vi "MakeTopFolder.vi"(8 "error in (no error)":errorcluster, 10 "Comment":string, 11 "Loggers":path=path "C:/Users/dpl/OneDrive - Aberystwyth University/Documents/LabVIEW Data/TestExecutive/TestData") -> (0 "error out":errorcluster, 2 "TopFolderPrefix":string, 3 "TestFolderPath":path)   [LabVIEW 2024]
uses:
  <userlib>/_OpenG.lib/file/file.llb/openg_file.lvlib
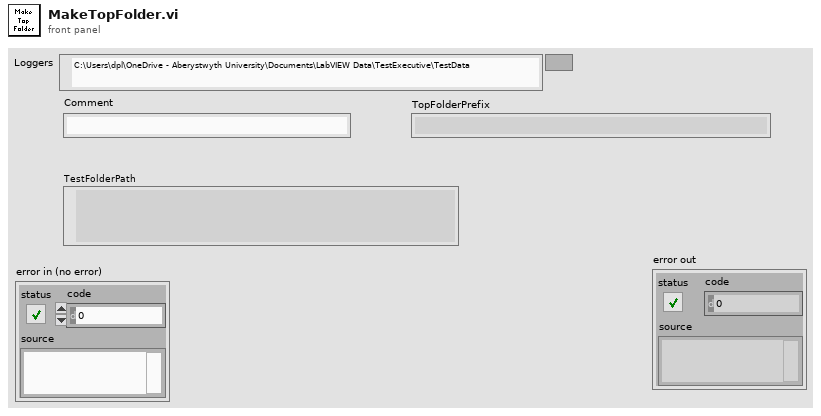
[diagram p1: front panel]
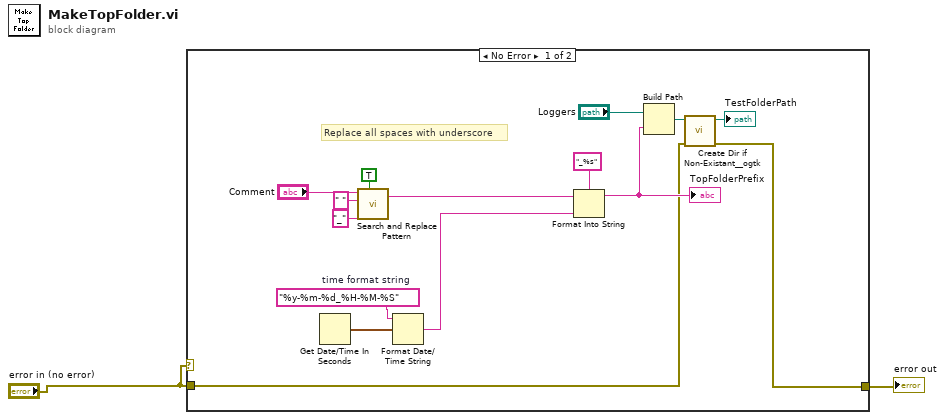
[diagram p0: block diagram]
diagram:
  n1 = case shown="No Error" "error in (no error)" {
    tunnel: "error in (no error)" -> [w4 w18]
    tunnel: [w3 w18] -> w1
    frame No Error {
      w16 = "%y-%m-%d_%H-%M-%S"  # time format string
      # "Replace all spaces with underscore"
      n2 = Get Date/Time In Seconds() -> (seconds since 1Jan1904=w17:timestamp)
      n3 = call <vilib>:"Search and Replace Pattern.vi"("string"="Comment", "regular expression (\"\")"=" " ("regular expression (\"\")"), "replace string (\"\")"="_" ("replace string (\"\")"), "replace all? (F)"=TRUE) -> ("result string"=w12:string)  [unwired: 1 in, 1 out]
      n4 = Format Date/Time String(time format string (%c)=w16, seconds (now)=w17) -> (date/time string=w14:string)  [unwired: 1 in]
      n5 = Format Into String(format string="_%s", initial string=w12, w14) -> (resulting string=w7:string)  [unwired: 1 in, 1 out]
      "TopFolderPrefix" <- w7
      n6 = Build Path(base path="Loggers", name or relative path=w7) -> (appended path=w8:path)
      n7 = call <userlib>:"Create Dir if Non-Existant__ogtk.vi"("error in (no error)"=w4, "Directory Path"=w8) -> ("error out"=w3:errorcluster, "dup Directory Path"=→"TestFolderPath":path)  [unwired: 7 in, 1 out]
    }
    frame Error {
    }
  }
  "error out" <- w1
